vi "format_time_lua.vi"(5 "LuaVIEW reference":T1) -> (15 "error out":errorcluster)   [LabVIEW 2012]
doc: "Uses the LabVIEW \"Format Date/Time String\" function to convert a numerical timestamp into a display string. See the LabVIEW documentation for information on how to construct a time format string.\n\nBEWARE: when daylight savings is enabled, the resulting date/time will jump by one hour twice a year. When you require a continously changing textual representation of time and do not mind it to being off by one hour for half the year, you may wish to disable daylight savings. Under Windows, this can be done via the timezone tab of the \"Date/Time\" control panel. Under Linux, this can be done by selecting a GMT+/-N timezone to fix the GMT offset.\nParameters:\nnum:time, number of seconds since the LabVIEW epoch.\n[str:format], when no format string is specified the format specified in the \"time format\" global is used.\nResults:\nstr:formatted_time"
uses:
  typedefs/t_LuaVIEW Reference.ctl
  subvis/private/LuaVIEW Pull (number).vi
  subvis/private/LuaVIEW Push (string).vi
  subvis/private/LuaVIEW Pull (string).vi
  library/glb_Library Configuration Globals.vi
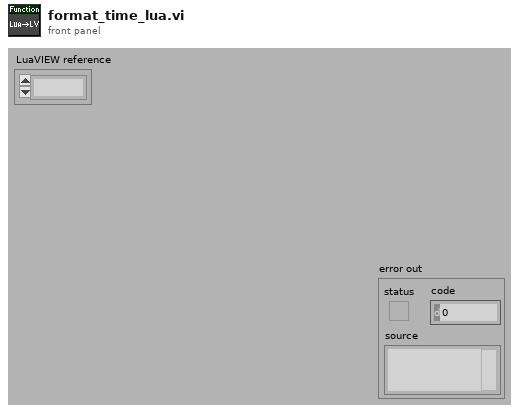
[diagram p1: front panel]
types:
  T1 = typedef "t_LuaVIEW Reference.ctl" = refnum<k1>
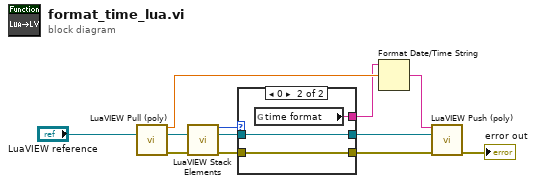
[diagram p0: block diagram]
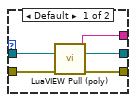
[diagram p2: hidden frame]
diagram:
  n1 = call-poly "LuaVIEW Pull (poly).vi"("LuaVIEW reference in"="LuaVIEW reference") -> ("number"=w7:dbl, "LuaVIEW reference out"=w8:T1, "error out"=w9:errorcluster)  [unwired: 12 in]
  n2 = call "LuaVIEW Stack Elements.vi"("LuaVIEW reference in"=w8, "error in (no error)"=w9) -> ("elements"=w6:i32, "LuaVIEW reference out"=w3:T1, "error out"=w4:errorcluster)  [unwired: 11 in]
  n3 = case shown="0" w6 {
    tunnel: [w14 w20] -> w5
    tunnel: w4 -> [w17 w19]
    tunnel: w3 -> [w16 w18]
    tunnel: [w15 w19] -> w2
    tunnel: [w13 w18] -> w1
    frame Default {
      n4 = call-poly "LuaVIEW Pull (poly).vi"("LuaVIEW reference in"=w16, "error in (no error)"=w17) -> ("string"=w14:string, "LuaVIEW reference out"=w13:T1, "error out"=w15:errorcluster)  [unwired: 11 in]
    }
    frame 0 {
      n5 = global read "glb_Library Configuration Globals.vi" "time format"() -> (w20:string)
    }
  }
  n6 = Format Date/Time String(time format string (%c)=w5, seconds (now)=w7) -> (date/time string=w12:string)  [unwired: 1 in]
  n7 = call-poly "LuaVIEW Push (poly).vi"("string"=w12, "LuaVIEW reference in"=w1, "error in (no error)"=w2) -> ("error out"=→"error out":errorcluster)  [unwired: 11 in, 1 out]
